vi "InitialisemyRIOFPGA.vi"() -> (0 "error out":errorcluster, 3 "Refnum out":refnum<k20>)   [LabVIEW 2019]
uses:
  <vilib>/FPGAPlugInAG/myRIO-1900/niLvFpga_Open_myRIO-1900.vi
  <vilib>/rvi/interface/common/dynamic/niFpgaDynamicAddResources.vi
  <vilib>/FPGAPlugInAG/Dynamic/niLvFpga_Reset_Dynamic.vi
  <vilib>/rvi/interface/common/niFpgaWaitOnOcc.vi
  <vilib>/Utility/error.llb/Error Cluster From Error Code.vi
  <vilib>/rvi/errors/niLvFpgaAdjustHostInterfaceError.vi
  <vilib>/FPGAPlugInAG/Dynamic/niLvFpga_Run_Dynamic.vi
  <vilib>/rvi/interface/nirviOpenFPGA/nirviOpenFPGA.xnode
  FPGA Bitfiles/RemoteTester_FPGATarget_FFT(FPGA)_Ir79AMG9Uqc.lvbitx
  <vilib>/rvi/interface/nirviMethod/nirviMethod.xnode
  <vilib>/rvi/interface/nirviReadWriteControl/nirviReadWriteControl.xnode
  NiFpgaLv.dll
  <vilib>/rvi/interface/Simulation/niFpgaSimulationCallBeginRW.vi
  <vilib>/FPGAPlugInAG/Dynamic/niLvFpga_ConfigureFifo_Dynamic.vi
  <vilib>/rvi/errors/niLvFpgaMergeErrorWithErrorCode.vi
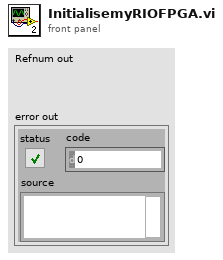
[diagram p1: front panel]
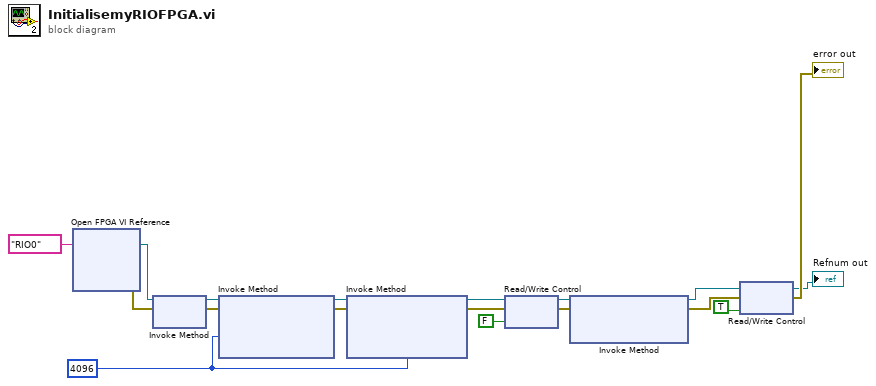
[diagram p0: block diagram]
diagram:
  w13 = u32 4096 ("Requested Depth")
  n1 = xnode "Open FPGA VI Reference"("resource name"=tag "RIO0") -> ("FPGA VI Reference Out"=w1:refnum<k20>, "error out"=w2:errorcluster)  [unwired: 1 in]
  n2 = xnode "Invoke Method"("FPGA VI Reference In"=w1, "error in"=w2) -> ("FPGA VI Reference Out"=w6:refnum<k20>, "error out"=w7:errorcluster)
  n3 = xnode "Invoke Method"("FPGA VI Reference In"=w6, "error in"=w7, "Requested Depth"=w13) -> ("FPGA VI Reference Out"=w8:refnum<k20>, "error out"=w9:errorcluster)  [unwired: 1 out]
  n4 = xnode "Invoke Method"("FPGA VI Reference In"=w8, "error in"=w9, "Requested Depth"=w13) -> ("FPGA VI Reference Out"=w10:refnum<k20>, "error out"=w11:errorcluster)  [unwired: 1 out]
  n5 = xnode "Read/Write Control"("FPGA VI Reference In"=w10, "error in"=w11, "stop"=FALSE) -> ("FPGA VI Reference Out"=w4:refnum<k20>, "error out"=w3:errorcluster)
  n6 = xnode "Invoke Method"("FPGA VI Reference In"=w4, "error in"=w3) -> ("FPGA VI Reference Out"=w15:refnum<k20>, "error out"=w17:errorcluster)  [unwired: 1 in]
  n7 = xnode "Read/Write Control"("FPGA VI Reference In"=w15, "error in"=w17, "LED0"=TRUE) -> ("FPGA VI Reference Out"=→"Refnum out":refnum<k20>, "error out"=→"error out":errorcluster)
